vi "ListboxStimulusAndAssert_Tests.vi"(11 "error in (no error)":errorcluster) -> (15 "error out":errorcluster)   [LabVIEW 2016, in "DronaTest.lvlib"]
uses:
  DronaTest.lvlib
  APIs/Stimulus/ControlValue/ValueSignalByPathString.vi
  APIs/Stimulus/ControlValue/SetValueAuto.vi
  APIs/Stimulus/ControlValue/ValueSignalLatchBooleanString.vi
  APIs/Assert/AssertControlValue/Equal.vi
  APIs/Assert/AssertControlValue/NotEqual.vi
  APIs/Assert/AssertSubpanel/AssertSubpanelVI.vi
  <vilib>/addons/_JKI Toolkits/Caraya/classes/Test/Test.lvclass
  Drona.lvlib
  APIs/Assert/AssertControlValue/AssertControlValue.lvlib
  APIs/Stimulus/ControlValue/ControlValue.lvlib
  APIs/Assert/AssertSubpanel/AssertSubpanel.lvlib
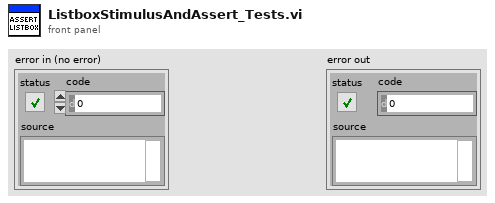
[diagram p1: front panel]
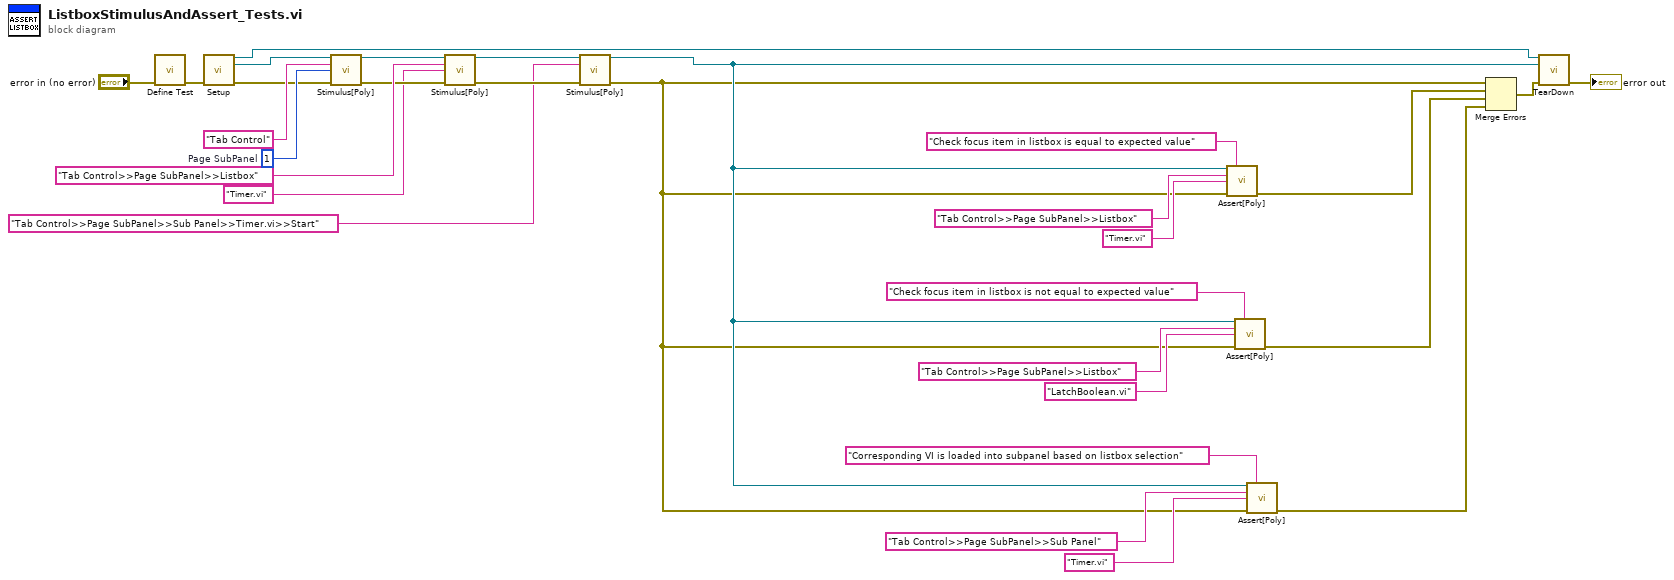
[diagram p0: block diagram]
diagram:
  w24 = 1  # Page SubPanel
  n1 = call <vilib>:"Define Test.vi"("error in (no error)"="error in (no error)") -> ("error out"=w29:errorcluster)  [unwired: 10 in]
  n2 = call "Setup.vi"("error in (no error)"=w29) -> ("Application Ref"=w26:refnum<vi>, "VI out"=w20:refnum<vi>, "error out"=w19:errorcluster)  [unwired: 12 in]
  n3 = call-poly "Stimulus[Poly].vi"("VI Reference In"=w20, "Control Path"="Tab Control", "Value (Signaling)"=w24, "error in"=w19) -> ("VI Reference Out"=w21:refnum<vi>, "error out"=w22:errorcluster)  [unwired: 10 in]
  n4 = call-poly "Stimulus[Poly].vi"("VI Reference In"=w21, "Control Path"="Tab Control>>Page SubPanel>>Listbox", "Value (Signaling)"="Timer.vi" ("Panel Name"), "error in"=w22) -> ("VI Reference Out"=w16:refnum<vi>, "error out"=w17:errorcluster)  [unwired: 10 in]
  n5 = call-poly "Stimulus[Poly].vi"("VI Reference In"=w16, "Control Path"="Tab Control>>Page SubPanel>>Sub Panel>>Timer.vi>>Start", "error in"=w17) -> ("VI Reference Out"=w6:refnum<vi>, "error out"=w3:errorcluster)  [unwired: 11 in]
  n6 = call-poly "Assert[Poly].vi"("VI Reference In"=w6, "Test Label"="Check focus item in listbox is equal to expected value", "Control Path"="Tab Control>>Page SubPanel>>Listbox", "Control Value"="Timer.vi" ("Panel Name"), "Error In"=w3) -> ("Error Out"=w11:errorcluster)  [unwired: 9 in, 1 out]
  n7 = call-poly "Assert[Poly].vi"("VI Reference In"=w6, "Test Label"="Check focus item in listbox is not equal to expected value", "Control Path"="Tab Control>>Page SubPanel>>Listbox", "Control Value"="LatchBoolean.vi" ("Panel Name"), "Error In"=w3) -> ("Error Out"=w8:errorcluster)  [unwired: 9 in, 1 out]
  n8 = call-poly "Assert[Poly].vi"("VI Reference In"=w6, "Test Label"="Corresponding VI is loaded into subpanel based on listbox selection", "Control Path"="Tab Control>>Page SubPanel>>Sub Panel", "VI Name"="Timer.vi" ("Panel Name"), "Error In"=w3) -> ("Error Out"=w2:errorcluster)  [unwired: 9 in, 1 out]
  n9 = Merge Errors(w3, w11, w8, w2) -> (w28:errorcluster)
  n10 = call "TearDown.vi"("Application Ref"=w26, "VI in"=w6, "error in (no error)"=w28) -> ("error out"=→"error out":errorcluster)  [unwired: 12 in]
